vi "Watchdog Reset.vi"(8 "error in":errorcluster, 11 "IED in":refnum<class "IED.lvclass">) -> (0 "error out":errorcluster, 3 "IED out":refnum<class "IED.lvclass">)   [LabVIEW 2018, in "IED Actor.lvlib" / "IED.lvclass"]
doc: "Publishes a DDS message to kick the watchdog of the current microgrid."
uses:
  IED.lvclass
  C:/Users/Administrator/Desktop/2018LabVIEW EMS/EMS Generic Actor/EMS Generic/EMS Generic.lvclass
  C:/Users/Administrator/Desktop/2018LabVIEW EMS/IED Actors/Device DDS Communications Framework/Device DDS Communications/Device DDS Communications.lvclass
  <vilib>/ORNL/CSEISMIC DDS/CSEISMIC DDS Base/Data Types/IED_watchdogReset.ctl
  Device DDS Communications Framework/Device DDS Communications/Device DDS Communications.lvclass/Device DDS Communications.ctl
  <vilib>/ORNL/CSEISMIC DDS/CSEISMIC DDS Base/CSEISMIC DDS.lvclass/CSEISMIC DDS.ctl
  <vilib>/ORNL/CSEISMIC DDS/CSEISMIC DDS Base/Accessors/Read DDS Reference.vi
  <vilib>/ORNL/CSEISMIC DDS/DDS Writer/DDS Writer.lvclass
  C:/Program Files (x86)/National Instruments/LabVIEW 2018/vi.lib/ORNL/CSEISMIC DDS/CSEISMIC DDS Base/CSEISMIC DDS.lvclass
  <vilib>/ORNL/CSEISMIC DDS/CSEISMIC DDS Base/Error Handler.vi
  <vilib>/ORNL/CSEISMIC DDS/CSEISMIC DDS Base/CSEISMIC DDS.lvclass
  Device DDS Communications Framework/Device DDS Communications/Device DDS Communications.lvclass
  EMS Generic Actor/EMS Generic/EMS Generic.lvclass
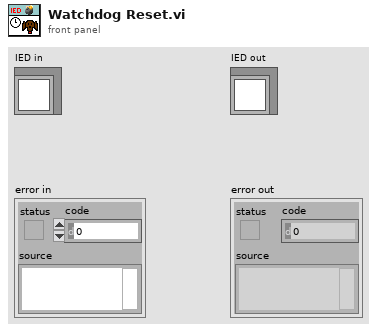
[diagram p1: front panel]
types:
  T1 = typedef "CSEISMIC DDS.lvlib/CSEISMIC DDS.lvclass/IED_watchdogReset.ctl" = cluster{"MicrogridID":u8}
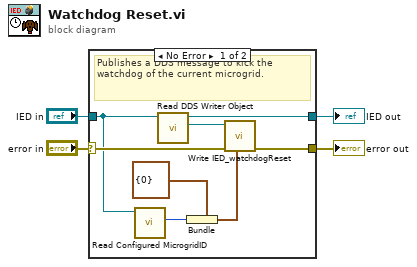
[diagram p0: block diagram]
diagram:
  n1 = case shown="No Error" "error in" {
    selector: "error in" -> [w9 w14]
    tunnel: [w8 w14] -> w3
    tunnel: [w5 w13] -> w1
    tunnel: "IED in" -> [w6 w13]
    frame No Error {
      # "Publishes a DDS message to kick the watchdog of the current microgrid."
      n2 = call "Read Configured MicrogridID.vi"("EMS Generic in"=w6) -> ("Microgrid ID"=w12:u8)  [unwired: 8 in, 2 out]
      n3 = call "Read DDS Writer Object.vi"("Device DDS Communications in"=w6) -> ("DDS Writer Object"=w10:refnum<class "DDS Writer.lvclass">, "Device DDS Communications out"=w5:refnum<class "IED.lvclass">)  [unwired: 9 in]
      n4 = Bundle(cluster=T1 {"MicrogridID"=0} ("Cluster"), "MicrogridID"=w12) -> (w7:T1)
      n5 = call <vilib>:"Write IED_watchdogReset.vi"("IED_watchdogReset"=w7, "error in"=w9, "DDS Writer in"=w10) -> ("error out"=w8:errorcluster)  [unwired: 7 in, 1 out]
    }
    frame Error {
    }
  }
  "error out" <- w3
  "IED out" <- w1
